vi "表格至数组.vi"(10 "表格控件":string[][](table)) -> (2 "数组":dbl[][](array[numeric]) format="%#.2f")   [LabVIEW 2010]
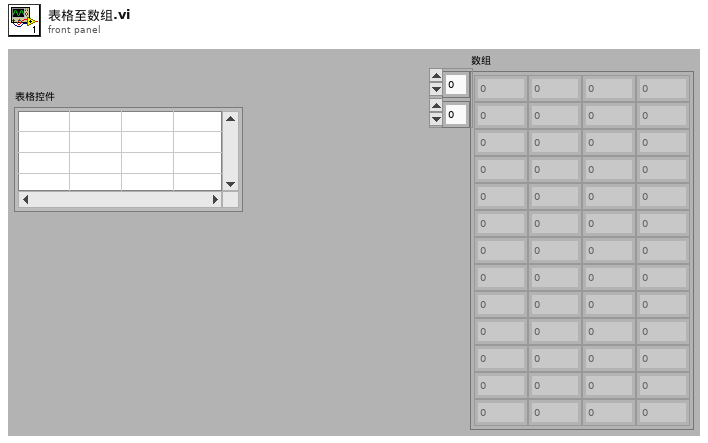
[diagram p1: front panel]
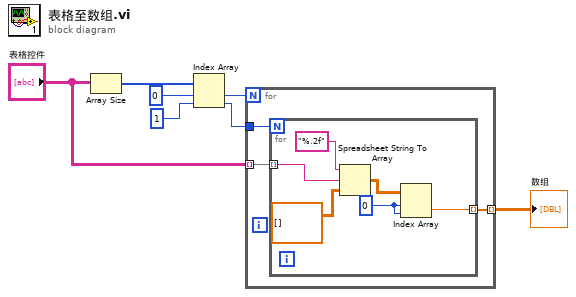
[diagram p0: block diagram]
diagram:
  n1 = Array Size(array="表格控件") -> (size(s)=w7:i32[])
  n2 = Index Array(array=w7, index #1=0 ("索引"), index #2=1 ("索引")) -> (element #1=w4:i32, element #2=w3:i32)
  n3 = for {
    N: w4 -> [_]
    tunnel: w3 -> [w10]
    tunnel: "表格控件" -> [w9] mode=indexing
    tunnel: [w8] -> w1 mode=indexing
    n4 = for {
      N: w10 -> [_]
      tunnel: w9 -> [w15] mode=indexing
      tunnel: [w11] -> w8 mode=indexing
      w12 = 0 ("索引 (行)")
      n5 = Spreadsheet String To Array(format string="%.2f" ("格式字符串"), spreadsheet string=w15, array type (2D Dbl)=dbl[][] [] ("数组类型(2D Dbl)")) -> (array=w13:dbl[][])  [unwired: 1 in]
      n6 = Index Array(array=w13, index (row)=w12, index (col)=w12) -> (element=w11:dbl)
    }
  }
  "数组" <- w1
